vi "getAdditionalDataFromXMLNative.vi"(8 "error in (no error)":errorcluster, 10 "eventXML":refnum<k20>, 11 "SingleToneRamp in":refnum<class "SingleToneRamp.lvclass">) -> (0 "error out":errorcluster, 2 "eventXML out":refnum<k20>, 3 "SingleToneRamp out":refnum<class "SingleToneRamp.lvclass">)   [LabVIEW 2011, in "Tools.lvlib" / "Scripting.lvlib" / "SingleToneRamp.lvclass"]
uses:
  SingleToneRamp.lvclass
  SingleToneRamp.lvclass/SingleToneRamp.ctl
  <vilib>/xml/Close Reference(Node).vi
  <vilib>/xml/NI_XML.lvlib
  SingleTone.lvclass
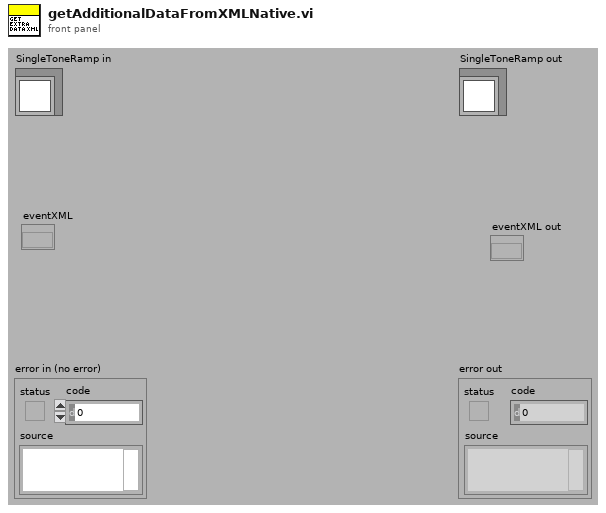
[diagram p1: front panel]
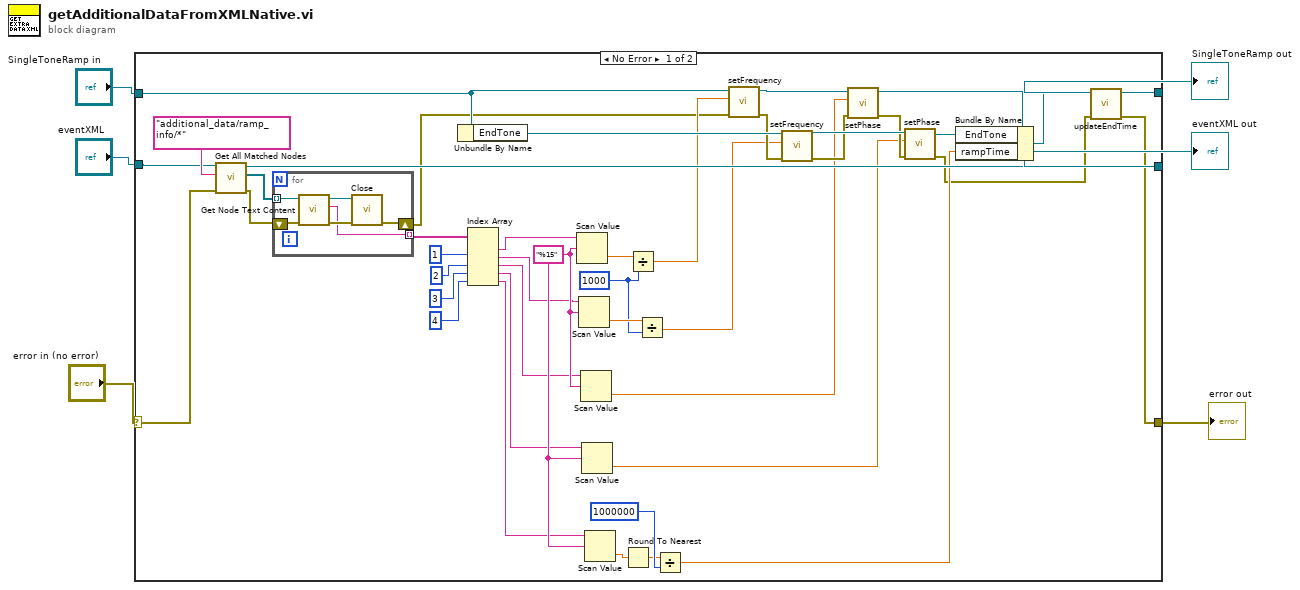
[diagram p0: block diagram]
diagram:
  n1 = case shown="No Error" "error in (no error)" {
    selector: "error in (no error)" -> [w43 w55]
    tunnel: [w8 w55] -> w1
    tunnel: "SingleToneRamp in" -> [w17 w56]
    tunnel: [w10 w56] -> w3
    tunnel: [w42 _] -> w2
    tunnel: "eventXML" -> [w41 _]
    frame No Error {
      w38 = 1000
      w37 = "%15"
      n2 = call <vilib>:"Get All Matched Nodes.vi"("error in (no error)"=w43, "XPath expression"="additional_data/ramp_info/*", "node in"=w41) -> ("error out"=w48:errorcluster, "node result array"=w46:refnum<k20>[], "node out"=w42:refnum<k20>)  [unwired: 6 in]
      n3 = for {
        tunnel: w46 -> [w51] mode=indexing
        tunnel: [w50] -> w45 mode=indexing
        shift-right: [w49] -> w15
        shift-left: w48 -> [w52]
        n4 = call <vilib>:"Get Node Text Content.vi"("error in (no error)"=w52, "node in"=w51) -> ("error out"=w53:errorcluster, "node text"=w50:string, "node out"=w54:refnum<k20>)  [unwired: 7 in]
        n5 = call-poly <vilib>:"Close.vi"("error in (no error)"=w53, "node"=w54) -> ("error out"=w49:errorcluster)  [unwired: 7 in]
      }
      n6 = Unbundle By Name(w17) -> ("EndTone"=w26:refnum<class "SingleTone.lvclass">)
      n7 = Index Array(array=w45, index #2=1 ("index"), index #3=2 ("index"), index #4=3 ("index"), index #5=4 ("index")) -> (element #1=w31:string, element #2=w30:string, element #3=w29:string, element #4=w28:string, element #5=w27:string)  [unwired: 1 in]
      n8 = Scan Value(string=w31, format string=w37) -> (value=w40:dbl)  [unwired: 1 in, 1 out]
      n9 = Scan Value(string=w30, format string=w37) -> (value=w39:dbl)  [unwired: 1 in, 1 out]
      n10 = Scan Value(string=w29, format string=w37) -> (value=w13:dbl)  [unwired: 1 in, 1 out]
      n11 = Scan Value(string=w28, format string=w37) -> (value=w12:dbl)  [unwired: 1 in, 1 out]
      n12 = Scan Value(string=w27, format string=w37) -> (value=w36:dbl)  [unwired: 1 in, 1 out]
      n13 = Round To Nearest(number=w36) -> (nearest integer value=w7:dbl)
      n14 = Divide(x=w40, y=w38) -> (x/y=w16:dbl)
      n15 = Divide(x=w39, y=w38) -> (x/y=w14:dbl)
      n16 = Divide(x=w7, y=1000000) -> (x/y=w11:dbl)
      n17 = call "setFrequency.vi"("error in (no error)"=w15, "frequency"=w16, "SingleTone.lvclass in"=w17) -> ("error out"=w25:errorcluster, "SingleTone.lvclass out"=w24:refnum<class "SingleToneRamp.lvclass">)  [unwired: 7 in]
      n18 = call "setFrequency.vi"("error in (no error)"=w25, "frequency"=w14, "SingleTone.lvclass in"=w26) -> ("error out"=w22:errorcluster, "SingleTone.lvclass out"=w23:refnum<class "SingleTone.lvclass">)  [unwired: 7 in]
      n19 = call "setPhase.vi"("error in (no error)"=w22, "phase"=w13, "SingleTone.lvclass in"=w24) -> ("error out"=w21:errorcluster, "SingleTone.lvclass out"=w20:refnum<class "SingleToneRamp.lvclass">)  [unwired: 7 in]
      n20 = call "setPhase.vi"("error in (no error)"=w21, "phase"=w12, "SingleTone.lvclass in"=w23) -> ("error out"=w9:errorcluster, "SingleTone.lvclass out"=w19:refnum<class "SingleTone.lvclass">)  [unwired: 7 in]
      n21 = Bundle By Name(cluster=w20, "EndTone"=w19, "rampTime"=w11) -> (w18:refnum<class "SingleToneRamp.lvclass">)
      n22 = call-dynamic "updateEndTime.vi"("error in (no error)"=w9, "SingleToneRamp in"=w18) -> ("error out"=w8:errorcluster, "SingleToneRamp out"=w10:refnum<class "SingleToneRamp.lvclass">)  [unwired: 8 in]
    }
    frame Error {
    }
  }
  "error out" <- w1
  "SingleToneRamp out" <- w3
  "eventXML out" <- w2
